vi "Arduino_Initialization_GCFS.vi"(7 "error in":errorcluster) -> (0 "error out":errorcluster, 2 "Connection":bool, 3 "VISA Arduino":refnum<visa-resource-name>)   [LabVIEW 2024]
uses:
  <vilib>/Instr/_visa.llb/VISA Find Search Mode.ctl
  <vilib>/Instr/_visa.llb/VISA Configure Serial Port (Instr).vi
  <vilib>/regexp/Match Regular Expression.xnode
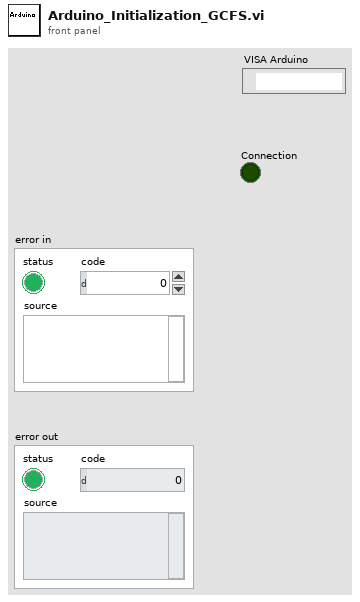
[diagram p1: front panel]
types:
  T1 = typedef "VISA Find Search Mode.ctl" = u32
  T2 = cluster{"VISA resource name out":refnum<visa-resource-name>, "error out":errorcluster}
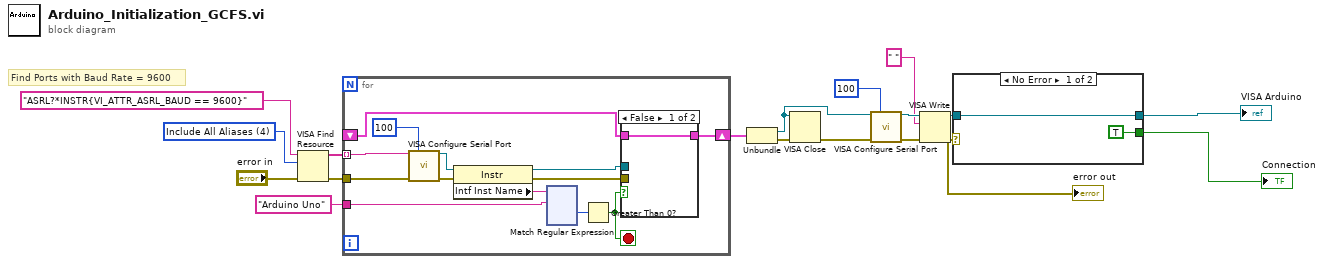
[diagram p0: block diagram]
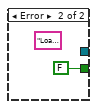
[diagram p2: hidden frame]
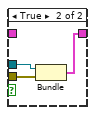
[diagram p3: hidden frame]
diagram:
  w6 = T1 4 items=["Canonical Names Only"=0, "Aliases Only"=2, "Include Matching Aliases"=3, "Include All Aliases"=4] ("Search Mode")
  # "Find Ports with Baud Rate = 9600"
  n1 = VISA Find Resource(8:"error in", 10:w6, 11:"ASRL?*INSTR{VI_ATTR_ASRL_BAUD == 9600}" ("expression (\"?*\")")) -> (0:w15:errorcluster, 3:w18:string[])  [unwired: 1 out]
  n2 = for {
    tunnel: w18 -> [w23] mode=indexing
    tunnel: "Arduino Uno" -> [w30]
    shift-right: [w29] -> w17
    shift-left: _ -> [w28]
    tunnel: w15 -> [w21]
    stop <- w24 stop-if-true
    n3 = call-poly "VISA Configure Serial Port"("VISA resource name"=w23, "timeout (10sec)"=u32 100 ("VISA Open timeout (0)"), "error in (no error)"=w21) -> ("VISA resource name out"=w22:refnum<visa-resource-name>, "error out"=w20:errorcluster)  [unwired: 11 in]
    n4 = property class="Instr"(reference=w22, error in=w20) -> (reference out=w27:refnum<visa-resource-name>, error out=w26:errorcluster, "Intf Inst Name"=w25:string)
    n5 = xnode "Match Regular Expression"("input string"=w25, "regular expression"=w30) -> ("offset past match"=w31:i32)  [unwired: 4 in, 4 out]
    n6 = Greater Than 0?(x=w31) -> (x > 0?=w24:bool)
    n7 = case shown="False" w24 {
      tunnel: w27 -> [_ w35]
      tunnel: w26 -> [_ w34]
      tunnel: [w32 w33] -> w29
      tunnel: w28 -> [w32 _]
      frame False {
      }
      frame True {
        n8 = Bundle("VISA resource name out"=w35, "error out"=w34) -> (w33:T2)  [unwired: 1 in]
      }
    }
  }
  n9 = Unbundle(w17) -> ("VISA resource name out"=w7:refnum<visa-resource-name>, "error out"=w12:errorcluster)
  n10 = VISA Close(VISA resource name=w7, error in (no error)=w12) -> (error out=w11:errorcluster)
  n11 = call-poly "VISA Configure Serial Port"("VISA resource name"=w7, "timeout (10sec)"=u32 100, "error in (no error)"=w11) -> ("VISA resource name out"=w10:refnum<visa-resource-name>, "error out"=w9:errorcluster)  [unwired: 11 in]
  n12 = VISA Write(VISA resource name=w10, write buffer=" ", error in (no error)=w9) -> (VISA resource name out=w5:refnum<visa-resource-name>, error out=w4:errorcluster)  [unwired: 1 out]
  "error out" <- w4
  n13 = case shown="No Error" w4 {
    tunnel: [TRUE FALSE] -> w1
    tunnel: w5 -> [w153 _]
    tunnel: [w153 _] -> w2
    frame No Error {
    }
    frame Error {
      (unwired) "Loading UI: Description >> MCU Connection Failed!\nUI: RTM >> TEMP_HIDE"
    }
  }
  "VISA Arduino" <- w2
  "Connection" <- w1
